vi "meth.ExecFunction.vi"(0 "GLue in":refnum<class "class.GLue.lvclass">, 2 "Name":string, 5 "Data in":variant, 11 "error in":errorcluster, 13 "ms timeout (-1)":i32=-1) -> (4 "GLue out":refnum<class "class.GLue.lvclass">, 6 "Data out":variant, 15 "error out":errorcluster)   [LabVIEW 2014, in "GLue.lvlib" / "class.GLue.lvclass"]
uses:
  class.GLue.lvclass
  class.GLue.lvclass/class.GLue.ctl
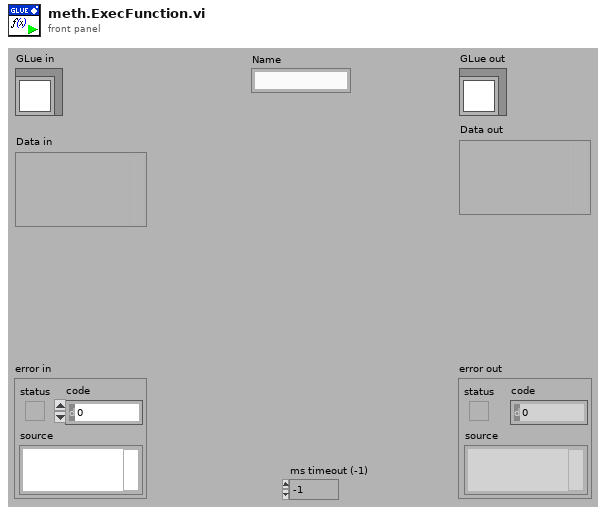
[diagram p1: front panel]
types:
  T1 = typedef "Semaphore RefNum" = refnum<k1>
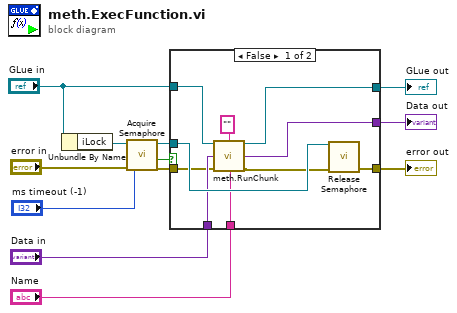
[diagram p0: block diagram]
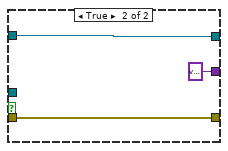
[diagram p2: hidden frame]
diagram:
  n1 = Unbundle By Name("GLue in") -> ("iLock"=w7:T1)
  n2 = call <vilib>:"Acquire Semaphore.vi"("error in (no error)"="error in", "ms timeout (-1)"="ms timeout (-1)", "semaphore"=w7) -> ("error out"=w5:errorcluster, "timed out"=w3:bool, "semaphore out"=w2:T1)  [unwired: 2 in]
  n3 = case shown="False" w3 {
    tunnel: [w22 w23] -> w12
    tunnel: [w19 w25] -> w11
    tunnel: "Name" -> [w14 _]
    tunnel: "Data in" -> [w17 _]
    tunnel: [w18 variant ("Data out")] -> w8
    tunnel: "GLue in" -> [w20 w25]
    tunnel: w5 -> [w16 w23]
    tunnel: w2 -> [w21 _]
    frame False {
      n4 = call "meth.RunChunk.vi"("GLue in"=w20, "Script"="", "Data in"=w17, "error in"=w16, "Name"=w14) -> ("GLue out"=w19:refnum<class "class.GLue.lvclass">, "Data out"=w18:variant, "error out"=w15:errorcluster)  [unwired: 8 in]
      n5 = call <vilib>:"Release Semaphore.vi"("error in (no error)"=w15, "semaphore"=w21) -> ("error out"=w22:errorcluster)  [unwired: 4 in, 1 out]
    }
    frame True {
    }
  }
  "error out" <- w12
  "GLue out" <- w11
  "Data out" <- w8
